vi "update.vi"(8 "error in (no error)":errorcluster, 11 "Analog_Output in":refnum<class "Analog_Output.lvclass">) -> (0 "error out":errorcluster, 3 "Analog_Output out":refnum<class "Analog_Output.lvclass">)   [LabVIEW 2013, in "Analog_Output.lvclass"]
uses:
  Analog_Output.lvclass
  Analog_Output.lvclass/Analog_Output.ctl
  <vilib>/DAQmx/write.llb/DAQmx Write (Analog 2D DBL NChan NSamp).vi
  Globals.vi
  <vilib>/DAQmx/configure/timing.llb/DAQmx Timing (Sample Clock).vi
  <vilib>/DAQmx/miscellaneous.llb/DAQmx Fill In Error Info.vi
panel:
  out "samples per channel":i32
  out "channels":i32
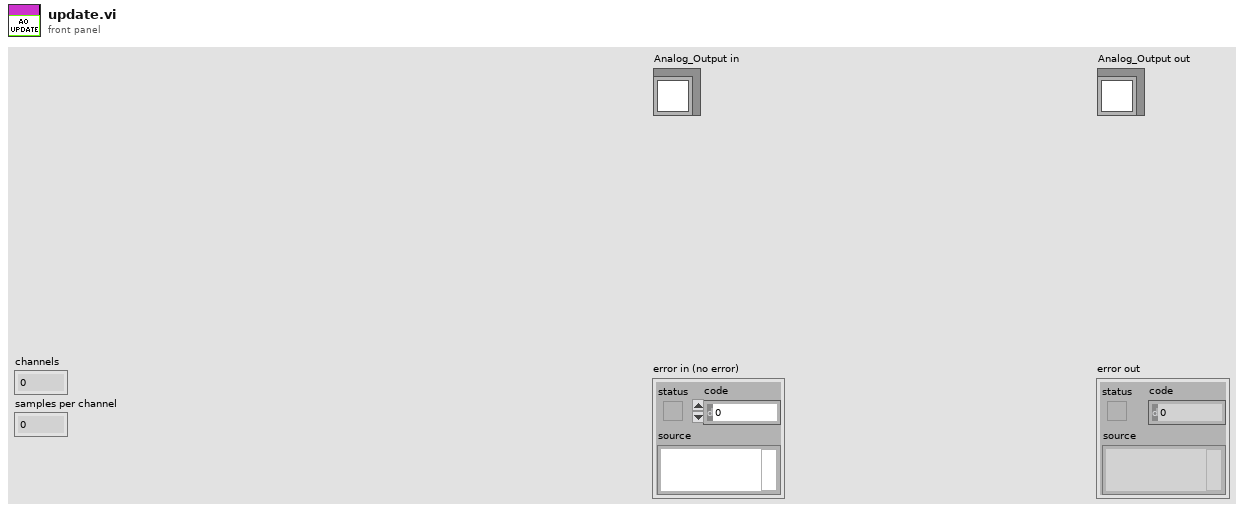
[diagram p1: front panel]
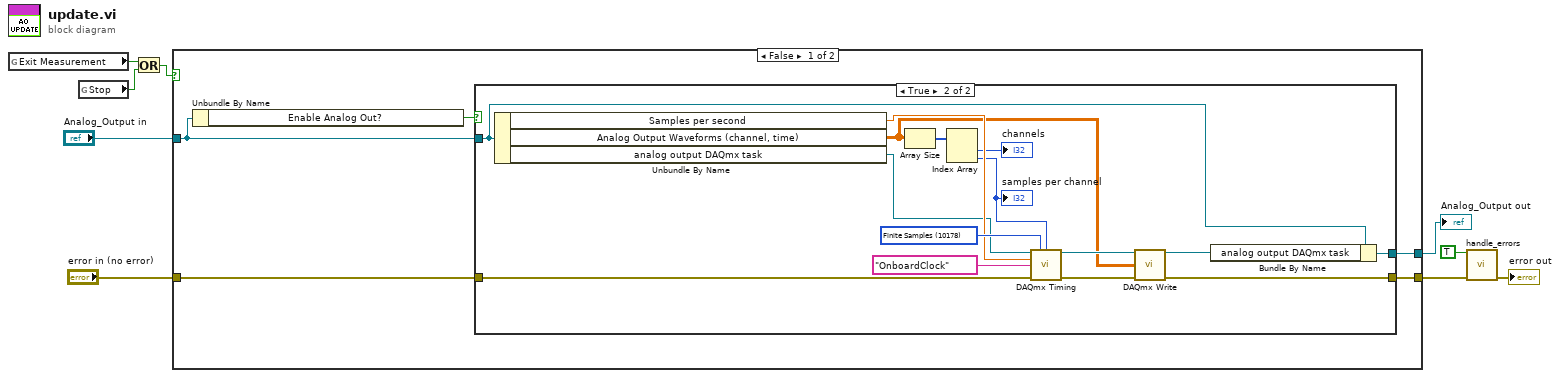
[diagram p0: block diagram]
diagram:
  n1 = global read "Globals.vi" "Exit Measurement"() -> (w7:bool)
  n2 = global read "Globals.vi" "Stop"() -> (w6:bool)
  n3 = Or(x=w7, y=w6) -> (x .or. y?=w5:bool)
  n4 = case shown="False" w5 {
    tunnel: [w14 w32] -> w3
    tunnel: [w12 w33] -> w8
    tunnel: "Analog_Output in" -> [w13 w33]
    tunnel: "error in (no error)" -> [w10 w32]
    frame False {
      n5 = Unbundle By Name(w13) -> ("Enable Analog Out?"=w11:bool)
      n6 = case shown="True" w11 {
        tunnel: w10 -> [w16 w20]
        tunnel: [w16 w31] -> w14
        tunnel: w13 -> [w15 w30]
        tunnel: [w15 w29] -> w12
        frame False {
        }
        frame True {
          w28 = 10178 items=["Finite Samples"=10178, "Continuous Samples"=10123, "Hardware Timed Single Point"=12522] ("sample mode")
          n7 = Unbundle By Name(w30) -> ("Samples per second"=w24:dbl, "Analog Output Waveforms (channel, time)"=w22:dbl[][], "analog output DAQmx task"=w19:refnum<k21>)
          n8 = Array Size(array=w22) -> (size(s)=w23:i32[])
          n9 = Index Array(array=w23) -> (element #1=→"channels":i32, element #2=w18:i32)  [unwired: 2 in]
          "samples per channel" <- w18
          n10 = call-poly <vilib>:"DAQmx Timing.vi"("task/channels in"=w19, "sample mode"=w28, "samples per channel"=w18, "rate"=w24, "source"=tag "OnboardClock", "error in"=w20) -> ("task out"=w27:refnum<k21>, "error out"=w25:errorcluster)  [unwired: 8 in]
          n11 = call-poly <vilib>:"DAQmx Write.vi"("task/channels in"=w27, "data"=w22, "error in"=w25) -> ("task out"=w21:refnum<k21>, "error out"=w31:errorcluster)  [unwired: 10 in, 1 out]
          n12 = Bundle By Name(cluster=w30, "analog output DAQmx task"=w21) -> (w29:refnum<class "Analog_Output.lvclass">)
        }
      }
    }
    frame True {
    }
  }
  "Analog_Output out" <- w8
  n13 = call "handle_errors.vi"("Exit Operation"=TRUE, "error in (no error)"=w3) -> ("error out"=→"error out":errorcluster)  [unwired: 13 in]
